vi "editTreeElement(Proj).vi"(8 "error in (no error)":errorcluster, 9 "Project File":string, 10 "Active Item:Tag":string, 11 "Tree Control in":refnum<vi>) -> (0 "error out":errorcluster)   [LabVIEW 2010]
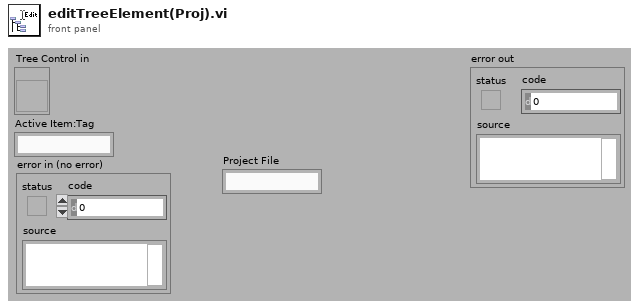
[diagram p1: front panel]
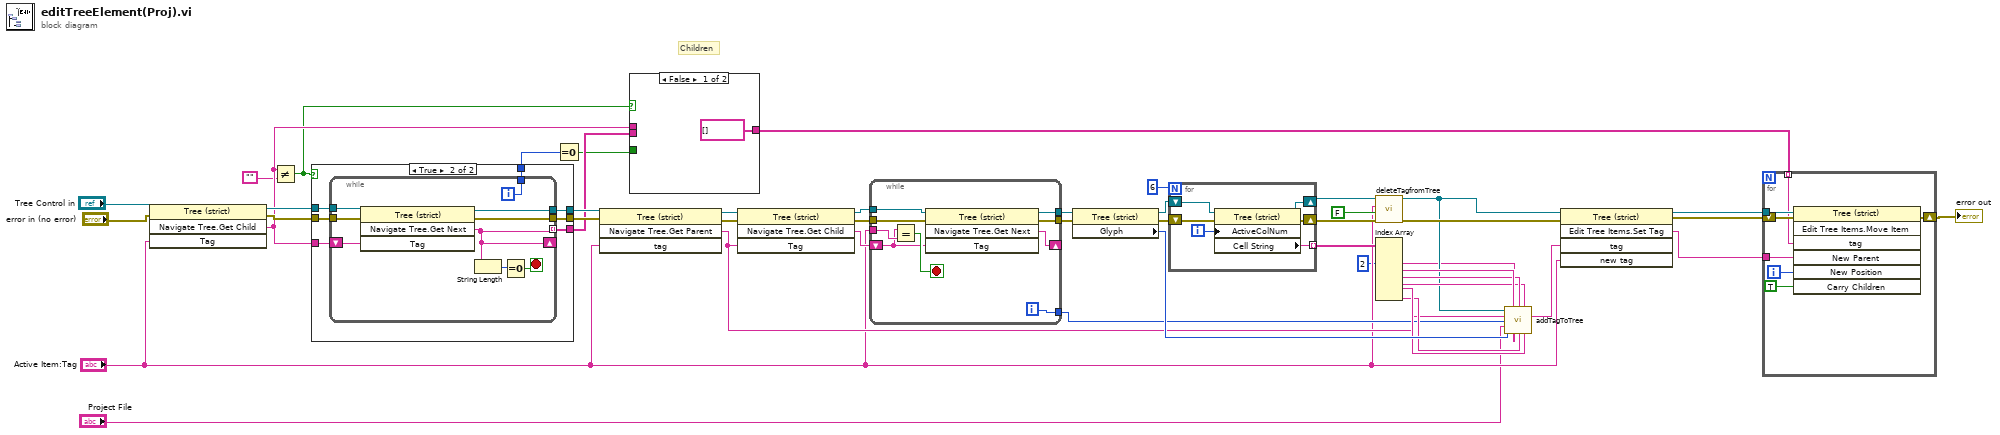
[diagram p0: block diagram]
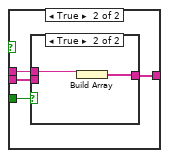
[diagram p2: hidden frame]
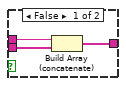
[diagram p3: hidden frame]
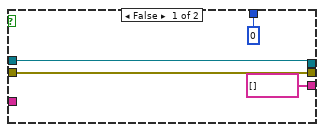
[diagram p4: hidden frame]
diagram:
  # "Children"
  n1 = invoke class="Tree (strict)" method="Navigate Tree.Get Child"(reference="Tree Control in", error in="error in (no error)", "Tag"="Active Item:Tag") -> (reference out=w18:refnum<vi>, error out=w17:errorcluster, "Navigate Tree:Get Child"=w6:string)  [unwired: 1 in, 1 out]
  n2 = Not Equal?(x=w6, y="") -> (x != y?=w4:bool)
  n3 = case shown="True" w4 {
    tunnel: w18 -> [w50 w57]
    tunnel: w17 -> [w49 w56]
    tunnel: [w50 w55] -> w16
    tunnel: [w49 w54] -> w15
    tunnel: [string[] [] w53] -> w14
    tunnel: [0 w52] -> w7
    tunnel: w6 -> [_ w51]
    frame False {
    }
    frame True {
      n4 = while {
        tunnel: w57 -> [w66]
        shift-right: [w59] -> _
        shift-left: w51 -> [w65]
        tunnel: w56 -> [w64]
        tunnel: [w63] -> w54
        tunnel: [w62] -> w55
        tunnel: [w59] -> w53 mode=indexing
        tunnel: [w58] -> w52
        i -> [w58]
        stop <- w60 stop-if-true
        n5 = invoke class="Tree (strict)" method="Navigate Tree.Get Next"(reference=w66, error in=w64, "Tag"=w65) -> (reference out=w62:refnum<vi>, error out=w63:errorcluster, "Navigate Tree:Get Next Item"=w59:string)  [unwired: 1 in, 1 out]
        n6 = String Length(string=w59) -> (length=w61:i32)
        n7 = Equal To 0?(x=w61) -> (x = 0?=w60:bool)
      }
    }
  }
  n8 = Equal To 0?(x=w7) -> (x = 0?=w8:bool)
  n9 = invoke class="Tree (strict)" method="Navigate Tree.Get Parent"(reference=w16, error in=w15, "tag"="Active Item:Tag") -> (reference out=w24:refnum<vi>, error out=w26:errorcluster, "Navigate Tree:Get Parent"=w28:string)  [unwired: 1 in, 1 out]
  n10 = case shown="False" w4 {
    tunnel: w14 -> [_ w71]
    tunnel: [string[] [] w70] -> w9
    tunnel: w8 -> [_ w69]
    tunnel: w6 -> [_ w68]
    frame False {
    }
    frame True {
      n11 = case shown="True" w69 {
        tunnel: w68 -> [w74 w76]
        tunnel: w71 -> [w73 _]
        tunnel: [w72 w75] -> w70
        frame False {
          n12 = Build Array (concatenate)(w74, w73) -> (w72:string[])
        }
        frame True {
          n13 = Build Array(w76) -> (w75:string[])
        }
      }
    }
  }
  n14 = invoke class="Tree (strict)" method="Navigate Tree.Get Child"(reference=w24, error in=w26, "Tag"=w28) -> (reference out=w29:refnum<vi>, error out=w27:errorcluster, "Navigate Tree:Get Child"=w30:string)  [unwired: 1 in, 1 out]
  n15 = while {
    tunnel: "Active Item:Tag" -> [w85]
    tunnel: [w83] -> w31
    tunnel: w29 -> [w82]
    shift-right: [w81] -> _
    shift-left: w30 -> [w80]
    tunnel: w27 -> [w79]
    tunnel: [w78] -> w25
    tunnel: [w77] -> w23
    i -> [w83]
    stop <- w84 stop-if-true
    n16 = Equal?(x=w80, y=w85) -> (x = y?=w84:bool)
    n17 = invoke class="Tree (strict)" method="Navigate Tree.Get Next"(reference=w82, error in=w79, "Tag"=w80) -> (reference out=w77:refnum<vi>, error out=w78:errorcluster, "Navigate Tree:Get Next Item"=w81:string)  [unwired: 1 in, 1 out]
  }
  n18 = property class="Tree (strict)"(reference=w23, error in=w25) -> (reference out=w44:refnum<vi>, error out=w43:errorcluster, "Glyph"=w45:i32)
  n19 = for {
    N: 6 -> [_]
    tunnel: [w88] -> w41 mode=indexing
    shift-right: [w86] -> w22
    shift-left: w44 -> [w91]
    shift-right: [w87] -> w34
    shift-left: w43 -> [w90]
    i -> [w89]
    n20 = property class="Tree (strict)"(reference=w91, error in=w90, "ActiveColNum"=w89) -> (reference out=w86:refnum<vi>, error out=w87:errorcluster, "Cell String"=w88:string)
  }
  n21 = call "deleteTagfromTree.vi"("error in (no error)"=w34, "Delete Children?"=FALSE, "Tag"="Active Item:Tag", "Tree Ref"=w22) -> ("error out"=w35:errorcluster, "Tree ref out"=w33:refnum<vi>)  [unwired: 6 in]
  n22 = Index Array(array=w41, index #2=2 ("index")) -> (element #2=w1:string, element #3=w40:string, element #4=w39:string, element #5=w38:string, element #6=w37:string, element #7=w36:string)  [unwired: 6 in, 1 out]
  n23 = call "addTagToTree.vi"("Tree ref"=w33, "Element name"=w40, "Calibration path"=w39, "Stimulus path"=w38, "parent tag"=w28, "Child Position"=w31, "new tag"="Project File", "Symbol"=w45, "Req"=w1, "Req doc path"=w36, "Analysis script path"=w37) -> ("New Element Tag"=w32:string)  [unwired: 4 in]
  n24 = invoke class="Tree (strict)" method="Edit Tree Items.Set Tag"(reference=w33, error in=w35, "tag"=w32, "new tag"="Active Item:Tag") -> (reference out=w11:refnum<vi>, error out=w12:errorcluster, "Edit Tree Items:Set Tag"=w10:string)  [unwired: 1 in, 2 out]
  n25 = for {
    tunnel: w11 -> [w96]
    tunnel: w10 -> [w95]
    tunnel: w9 -> [w94] mode=indexing
    shift-right: [w98] -> w13
    shift-left: w12 -> [w97]
    i -> [w93]
    n26 = invoke class="Tree (strict)" method="Edit Tree Items.Move Item"(reference=w96, error in=w97, "tag"=w94, "New Parent"=w95, "New Position"=w93, "Carry Children"=TRUE ("Carry Children?")) -> (error out=w98:errorcluster)  [unwired: 1 in, 6 out]
  }
  "error out" <- w13
